vi "SPCM_Example.vi"() -> ()   [LabVIEW 2009]
panel:
  out "XY Graph":cluster{"Y":dbl[], "Y":dbl[]}[](graph)
  in  "Bins Per Array":u32
  in  "Pulse Blind Time [ns]":dbl format="%#_13g"
  in  "stop":bool
  out "Counts Value":i32
  in  "Bin Length [ms]":u32
  in  "Pause Time [ms]":dbl format="%#_13g"
  out "Device Name":string
  out "Serial Number":string
  # "SPCM Example\n\nOperating mode: Timer free running"
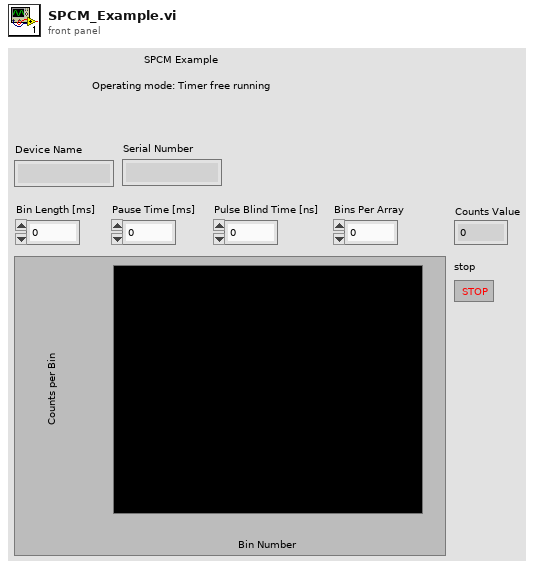
[diagram p1: front panel]
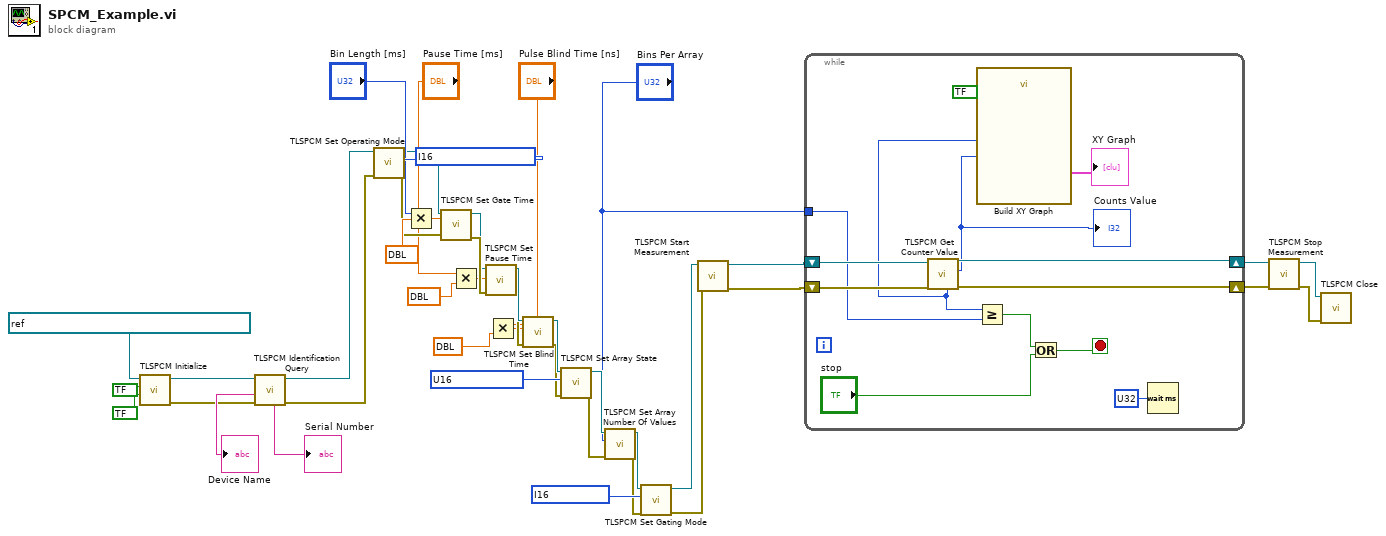
[diagram p0: block diagram]
diagram:
  w9 = i16 ? items=["APD Gating", "Counter Gating"] ("Gating Mode (Counter Gating)")
  w32 = i16 ? items=["User Mode", "Timer Free Running", "Triggered by Timer", "Triggered by external Signal", "Gating by External Signal"] ("Operating Mode (Triggered by Timer)")
  w35 = u16 ? items=["Array State Off", "Array State On"] ("Set Array State (Array State Off)")
  n1 = call "TLSPCM Initialize.vi"("Reset Device (Reset Device)"=bool ?, "ID Query (Do Query)"=bool ?, "resource name"=refnum<visa-resource-name> ?) -> ("error out"=w33:errorcluster, "instrument handle out"=w37:refnum<visa-resource-name>)  [unwired: 7 in]
  n2 = call "TLSPCM Identification Query.vi"("error in (no error)"=w33, "instrument handle"=w37) -> ("error out"=w34:errorcluster, "Device Name"=→"Device Name":string, "instrument handle out"=w36:refnum<visa-resource-name>, "Serial Number"=→"Serial Number":string)  [unwired: 4 in, 2 out]
  n3 = call "TLSPCM Set Operating Mode.vi"("error in (no error)"=w34, "Operating Mode (Triggered by Timer)"=w32, "instrument handle"=w36) -> ("error out"=w23:errorcluster, "instrument handle out"=w24:refnum<visa-resource-name>)  [unwired: 7 in]
  n4 = Multiply(x="Bin Length [ms]", y=dbl ?) -> (x*y=w27:dbl)
  n5 = call "TLSPCM Set Gate Time.vi"("error in (no error)"=w23, "Gate Time (0.1)"=w27, "instrument handle"=w24) -> ("error out"=w22:errorcluster, "instrument handle out"=w21:refnum<visa-resource-name>)  [unwired: 7 in]
  n6 = Multiply(x="Pause Time [ms]", y=dbl ?) -> (x*y=w20:dbl)
  n7 = call "TLSPCM Set Pause Time.vi"("error in (no error)"=w22, "Pause Time (0.000001)"=w20, "instrument handle"=w21) -> ("error out"=w16:errorcluster, "instrument handle out"=w17:refnum<visa-resource-name>)  [unwired: 7 in]
  n8 = Multiply(x="Pulse Blind Time [ns]", y=dbl ?) -> (x*y=w15:dbl)
  n9 = call "TLSPCM Set Blind Time.vi"("error in (no error)"=w16, "Blind Time (0.0)"=w15, "instrument handle"=w17) -> ("error out"=w12:errorcluster, "instrument handle out"=w13:refnum<visa-resource-name>)  [unwired: 7 in]
  n10 = call "TLSPCM Set Array State.vi"("error in (no error)"=w12, "Set Array State (Array State Off)"=w35, "instrument handle"=w13) -> ("error out"=w10:errorcluster, "instrument handle out"=w11:refnum<visa-resource-name>)  [unwired: 7 in]
  n11 = call "TLSPCM Set Array Number Of Values.vi"("error in (no error)"=w10, "Number of Array Values (100)"="Bins Per Array", "instrument handle"=w11) -> ("error out"=w7:errorcluster, "instrument handle out"=w8:refnum<visa-resource-name>)  [unwired: 7 in]
  n12 = call "TLSPCM Set Gating Mode.vi"("error in (no error)"=w7, "Gating Mode (Counter Gating)"=w9, "instrument handle"=w8) -> ("error out"=w5:errorcluster, "instrument handle out"=w6:refnum<visa-resource-name>)  [unwired: 7 in]
  n13 = call "TLSPCM Start Measurement.vi"("error in (no error)"=w5, "instrument handle"=w6) -> ("error out"=w4:errorcluster, "instrument handle out"=w3:refnum<visa-resource-name>)  [unwired: 8 in]
  n14 = while {
    shift-right: [w55] -> w31
    shift-left: w3 -> [w53]
    shift-right: [w54] -> w30
    shift-left: w4 -> [w52]
    tunnel: "Bins Per Array" -> [w46]
    stop <- w45 stop-if-true
    n15 = call "TLSPCM Get Counter Value.vi"("error in (no error)"=w52, "instrument handle"=w53) -> ("error out"=w54:errorcluster, "Counter"=w49:u32, "instrument handle out"=w55:refnum<visa-resource-name>, "Index of Counter"=w47:u32)  [unwired: 5 in, 1 out]
    "Counts Value" <- w49
    n16 = call "Build XY Graph"("Reset"=bool ?, "Y Input"=w49, "X Input"=w47) -> ("XY Graph"=→"XY Graph":cluster{"X":dbl[], "Y":dbl[]}[])  [unwired: 7 in, 1 out]
    n17 = Greater Or Equal?(x=w47, y=w46) -> (x >= y?=w44:bool)
    n18 = Or(x=w44, y="stop") -> (x .or. y?=w45:bool)
    n19 = Wait (ms)(milliseconds to wait=u32 ?) -> ()  [unwired: 1 out]
  }
  n20 = call "TLSPCM Stop Measurement.vi"("error in (no error)"=w30, "instrument handle"=w31) -> ("error out"=w29:errorcluster, "instrument handle out"=w28:refnum<visa-resource-name>)  [unwired: 8 in]
  n21 = call "TLSPCM Close.vi"("error in (no error)"=w29, "instrument handle"=w28) -> ()  [unwired: 9 in, 1 out]
